vi "Listen.vi"(8 "error in (no error)":errorcluster, 11 "TCP_Listener in":refnum<class "TCP_Listener.lvclass">) -> (0 "error out":errorcluster, 3 "TCP_Listener out":refnum<class "TCP_Listener.lvclass">)   [LabVIEW 2023, in "TCP_Listener.lvlib" / "TCP_Listener.lvclass"]
uses:
  TCP_Listener.lvclass
  C:/Program Files (x86)/National Instruments/LabVIEW 2023/vi.lib/ActorFramework/Actor/Actor.lvclass
  <vilib>/ActorFramework/Actor/Actor.lvclass/Actor.ctl
  <vilib>/ActorFramework/Message Enqueuer/Message Enqueuer.lvclass/Message Enqueuer.ctl
  TCP_Listener.lvclass/TCP_Listener.ctl
  TypeDefinitions/ConnectionInformation.ctl
  Connections Controller Messages/NewConnection Msg/NewConnection Msg.lvclass/NewConnection Msg.ctl
  <vilib>/ActorFramework/Message Enqueuer/Init from Existing Queue.vi
  <vilib>/ActorFramework/Message Enqueuer/Enqueue.vi
  Connections Controller Messages/NewConnection Msg/NewConnection Msg.lvclass
  C:/Program Files (x86)/National Instruments/LabVIEW 2023/vi.lib/ActorFramework/Message/Message.lvclass
  TCP_Listener Messages/Listen Msg/Listen Msg.lvclass
  <vilib>/ActorFramework/Stop Msg/Stop Msg.lvclass
  <vilib>/ActorFramework/Message Priority Queue/Priority Enqueue.vi
  <vilib>/ActorFramework/Message Enqueuer/Message Enqueuer.lvclass
  <vilib>/ActorFramework/Actor/Actor.lvclass
  TCP_Listener.lvlib
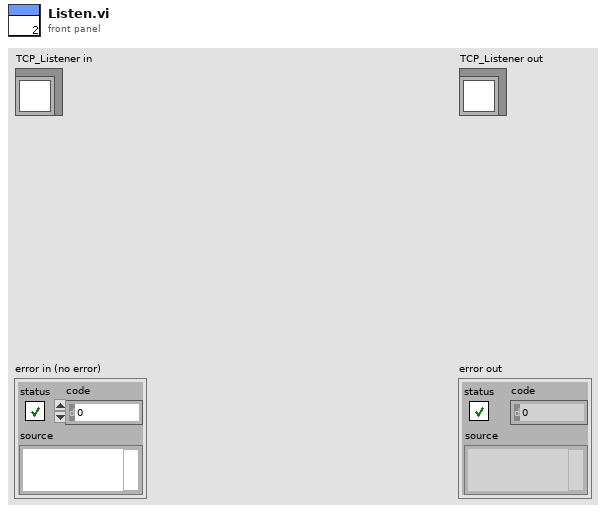
[diagram p1: front panel]
types:
  T1 = typedef "TCP_Listener.lvlib/ConnectionInformation.ctl" = cluster{"Connection number":i32, "Remote Address":string, "Remote Port":u16, "Connection ID":refnum<k5>}
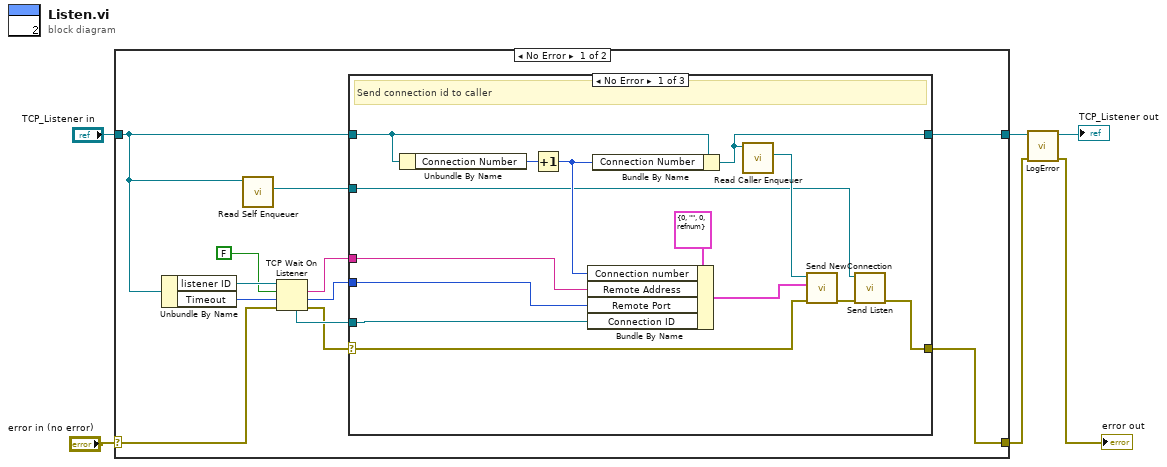
[diagram p0: block diagram]
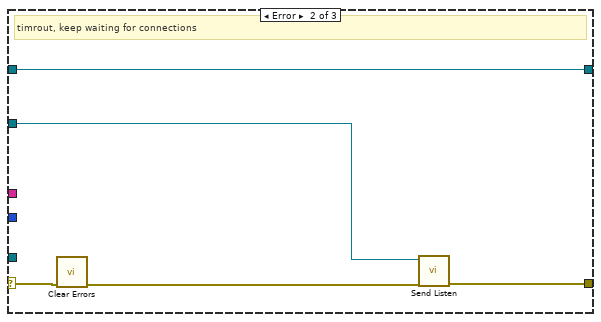
[diagram p2: hidden frame]
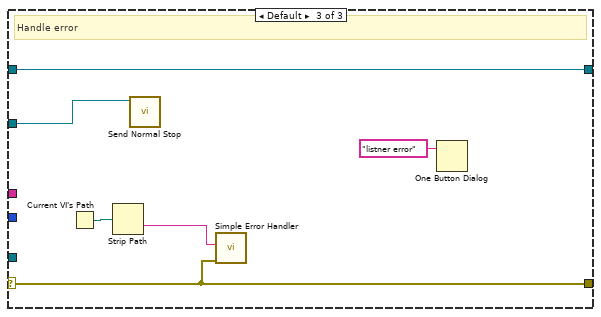
[diagram p3: hidden frame]
diagram:
  n1 = case shown="No Error" "error in (no error)" {
    selector: "error in (no error)" -> [w17 w45]
    tunnel: [w14 w45] -> w2
    tunnel: [w12 w44] -> w4
    tunnel: "TCP_Listener in" -> [w13 w44]
    frame No Error {
      n2 = Unbundle By Name(w13) -> ("listener ID"=w18:refnum<k5>, "Timeout"=w9:i32)
      n3 = call <vilib>:"Read Self Enqueuer.vi"("Actor"=w13) -> ("Self Enqueuer"=w11:refnum<class "Message Enqueuer.lvclass">)  [unwired: 10 in]
      n4 = TCP Wait On Listener(8:w17, 9:w9, 10:FALSE ("resolve remote address (T)"), 11:w18) -> (0:w7:errorcluster, 1:w15:u16, 2:w8:string, 4:w16:refnum<k5>)  [unwired: 1 out]
      n5 = case shown="No Error" w7 {
        selector: w7 -> [w26 w37 w41]
        tunnel: w16 -> [w28 _ _]
        tunnel: w8 -> [w30 _ _]
        tunnel: w15 -> [w29 _ _]
        tunnel: [w19 w35 w41] -> w14
        tunnel: w13 -> [w24 w36 w43]
        tunnel: [w22 w36 w43] -> w12
        tunnel: w11 -> [w20 w33 w42]
        frame No Error {
          # "Send connection id to caller"
          n6 = Unbundle By Name(w24) -> ("Connection Number"=w25:i32)
          n7 = Increment(x=w25) -> (x+1=w23:i32)
          n8 = Bundle By Name(cluster=T1 {"Connection number"=0, "Remote Address"="", "Remote Port"=0, "Connection ID"=refnum} ("Connection Information"), "Connection number"=w23, "Remote Address"=w30, "Remote Port"=w29, "Connection ID"=w28) -> (w27:T1)
          n9 = Bundle By Name(cluster=w24, "Connection Number"=w23) -> (w22:refnum<class "TCP_Listener.lvclass">)
          n10 = call <vilib>:"Read Caller Enqueuer.vi"("Actor"=w22) -> ("Caller Enqueuer"=w32:refnum<class "Message Enqueuer.lvclass">)  [unwired: 10 in]
          n11 = call "Send NewConnection.vi"("error in (no error)"=w26, "Connection Information"=w27, "Message Enqueuer"=w32) -> ("error out"=w21:errorcluster)  [unwired: 7 in, 1 out]
          n12 = call "Send Listen.vi"("error in (no error)"=w21, "Message Enqueuer"=w20) -> ("error out"=w19:errorcluster)  [unwired: 8 in, 1 out]
        }
        frame Error {
          # "timrout, keep waiting for connections"
          n13 = call <vilib>:"Clear Errors.vi"("error in (no error)"=w37) -> ("error out"=w34:errorcluster)  [unwired: 5 in, 1 out]
          n14 = call "Send Listen.vi"("error in (no error)"=w34, "Message Enqueuer"=w33) -> ("error out"=w35:errorcluster)  [unwired: 8 in, 1 out]
        }
        frame Default {
          # "Handle error"
          n15 = Current VI's Path() -> (path=w39:path)
          n16 = Strip Path(path=w39) -> (name=w38:string)  [unwired: 1 out]
          n17 = call <vilib>:"Send Normal Stop.vi"("Message Enqueuer"=w42) -> ()  [unwired: 10 in, 1 out]
          n18 = call <vilib>:"Simple Error Handler.vi"("error source (\" \")"=w38, "error in (no error)"=w41) -> ()  [unwired: 3 in, 5 out]
          n19 = One Button Dialog(message="listner error") -> ()  [unwired: 1 in, 1 out]
        }
      }
    }
    frame Error {
    }
  }
  n20 = call "LogError.vi"("error in (no error)"=w2, "TCP_Listener in"=w4) -> ("error out"=→"error out":errorcluster, "TCP_Listener out"=→"TCP_Listener out":refnum<class "TCP_Listener.lvclass">)  [unwired: 8 in]
